vi "ReferencePoints_PixelValue.vi"(11 "ItemNames":string[][](array[string])) -> (3 "Pixel Coordinates":cluster{dbl, dbl}[](array[cluster]))   [LabVIEW 2015]
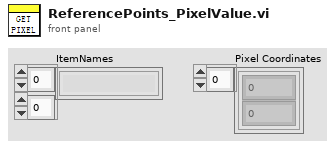
[diagram p1: front panel]
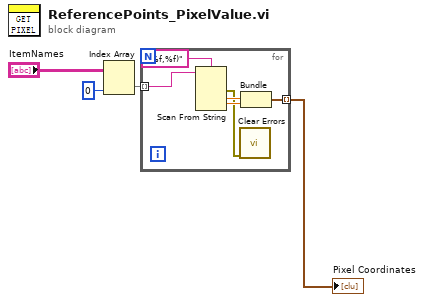
[diagram p0: block diagram]
diagram:
  n1 = Index Array(array="ItemNames", index (col)=0 ("disabled index (col)")) -> (element=w3:string[])  [unwired: 1 in]
  n2 = for {
    tunnel: w3 -> [w10] mode=indexing
    tunnel: [w6] -> w4 mode=indexing
    n3 = Scan From String(format string="(%f,%f)", input string=w10) -> (error out=w5:errorcluster, output 1=w8:dbl, output 2=w7:dbl)  [unwired: 4 in, 2 out]
    n4 = call <vilib>:"Clear Errors.vi"("error in (no error)"=w5) -> ()  [unwired: 5 in, 2 out]
    n5 = Bundle(w8, w7) -> (w6:cluster{dbl, dbl})  [unwired: 1 in]
  }
  "Pixel Coordinates" <- w4
